vi "FeetToTicks.vi"(11 "x":dbl=1.0) -> (3 "Numeric":dbl)   [LabVIEW 2017]
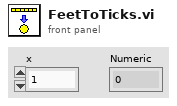
[diagram p1: front panel]
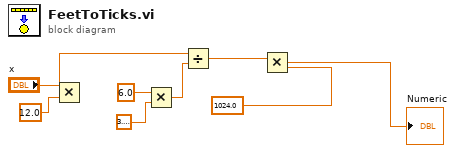
[diagram p0: block diagram]
diagram:
  n1 = Multiply(x="x", y=12.0) -> (x*y=w2:dbl)
  n2 = Multiply(x=6.0, y=3.141592653589793) -> (x*y=w5:dbl)
  n3 = Divide(x=w2, y=w5) -> (x/y=w6:dbl)
  n4 = Multiply(x=w6, y=1024.0) -> (x*y=→"Numeric":dbl)
